vi "A33Initialize_py.vi"(8 "error in (no error)":errorcluster, 10 "Instrument":string="AG33600A_Gen1", 11 "socket in":refnum<class "zmq_socket.lvclass">) -> (0 "error out":errorcluster, 1 "Standalone":bool, 2 "resulting string":string, 3 "socket out":refnum<class "zmq_socket.lvclass">)   [LabVIEW 2022 SP3]
doc: "Selects the waveform shape, frequency, amplitude, offset, and phase for a standard waveform."
uses:
  <vilib>/addons/zeromq/zmq_socket.lvclass
panel:
  in  "Reset":bool=TRUE
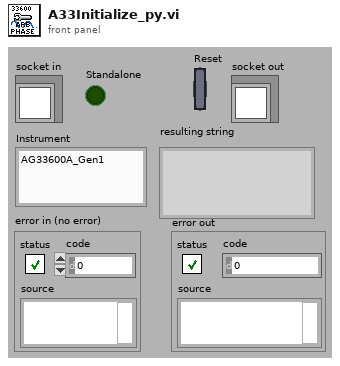
[diagram p1: front panel]
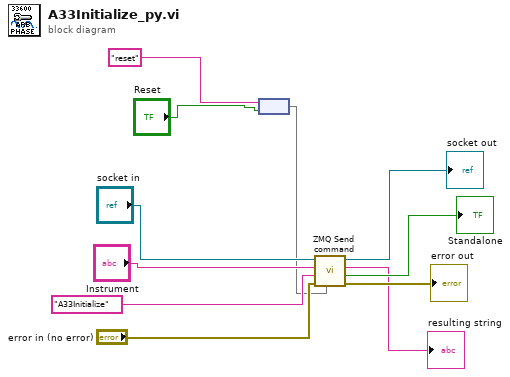
[diagram p0: block diagram]
diagram:
  n1 = node("reset" ("key"), "Reset") -> (w3:map{string, bool})
  n2 = call "ZMQ Send command.vi"("Bool args"=w3, "error in"="error in (no error)", "Command"="A33Initialize", "Instrument"="Instrument", "socket in"="socket in") -> ("error out"=→"error out":errorcluster, "Standalone"=→"Standalone":bool, "Recieved message"=→"resulting string":string, "socket out"=→"socket out":refnum<class "zmq_socket.lvclass">)  [unwired: 3 in]
